vi "InitialMove.vi"(8 "error in (no error)":errorcluster, 10 "SnakeGame in":refnum<class "SnakeGame.lvclass">, 11 "Snake in":refnum<class "Snake.lvclass">) -> (0 "error out":errorcluster, 2 "SnakeGame out":refnum<class "SnakeGame.lvclass">, 3 "Snake out":refnum<class "Snake.lvclass">)   [LabVIEW 2019, in "RT_Game.lvlib" / "Snake.lvclass"]
uses:
  Snake.lvclass
  SnakeGame/SnakeGame.lvclass
  Snake.lvclass/Snake.ctl
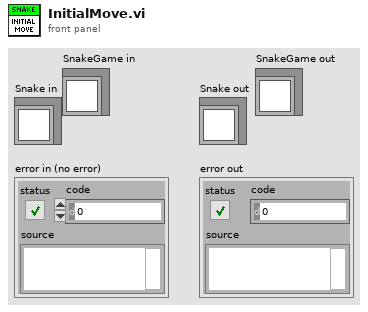
[diagram p1: front panel]
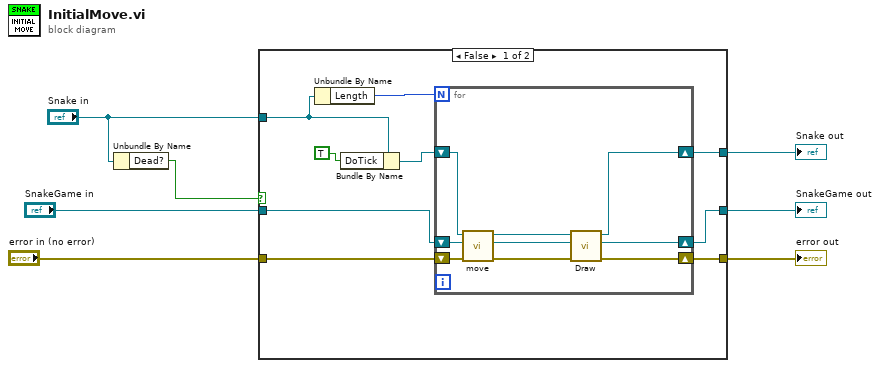
[diagram p0: block diagram]
diagram:
  n1 = Unbundle By Name("Snake in") -> ("Dead?"=w1:bool)
  n2 = case shown="False" w1 {
    tunnel: "Snake in" -> [w13 w28]
    tunnel: [w12 w28] -> w7
    tunnel: [w11 w26] -> w6
    tunnel: "error in (no error)" -> [w10 w26]
    tunnel: "SnakeGame in" -> [w9 w27]
    tunnel: [w8 w27] -> w3
    frame False {
      n3 = Unbundle By Name(w13) -> ("Length"=w14:i16)
      n4 = Bundle By Name(cluster=w13, "DoTick"=TRUE) -> (w15:refnum<class "Snake.lvclass">)
      n5 = for {
        N: w14 -> [_]
        shift-right: [w21] -> w11
        shift-left: w10 -> [w25]
        shift-right: [w19] -> w12
        shift-left: w15 -> [w23]
        shift-right: [w17] -> w8
        shift-left: w9 -> [w22]
        n6 = call "move.vi"("error in (no error)"=w25, "SnakeGame in"=w22, "Snake in"=w23) -> ("error out"=w24:errorcluster, "SnakeGame out"=w18:refnum<class "SnakeGame.lvclass">, "Snake out"=w20:refnum<class "Snake.lvclass">)  [unwired: 6 in]
        n7 = call "Draw.vi"("error in (no error)"=w24, "Snake in 2"=w18, "Snake in"=w20) -> ("error out"=w21:errorcluster, "Snake out 2"=w17:refnum<class "SnakeGame.lvclass">, "Snake out"=w19:refnum<class "Snake.lvclass">)  [unwired: 6 in]
      }
    }
    frame True {
    }
  }
  "Snake out" <- w7
  "error out" <- w6
  "SnakeGame out" <- w3
